vi "Quaternion_ToRotationVector.vi"(11 "Quaternion":T1={"R"=1.0, "V"=[0.0, 0.0, 0.0]}) -> (3 "RotationVector":dbl[](array[numeric]))   [LabVIEW 2019, in "Trajectory_Library.lvlib"]
doc: "Returns the rotation vector representation of this quaternion.\n\nThis is also the log operator of SO(3).\n\nParameters:\n - Quaternion -- The quaternion data cluster.\n\nReturns:\n - Rotation Vector - The rotation vector representation of this quaternion."
uses:
  Trajectory_Library.lvlib
  TypeDef/QUATERNION.ctl
  <vilib>/Analysis/_algsub.llb/Matrix Norm.vi
  <vilib>/Analysis/_algsub.llb/Real Matrix Norm.vi
  <vilib>/Analysis/Matrix/Numeric/Conversions/Array To Matrix - RA.vi
  <vilib>/Analysis/Matrix/NI_Matrix.lvlib
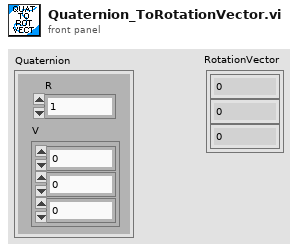
[diagram p1: front panel]
types:
  T1 = typedef "Trajectory_Library.lvlib/QUATERNION.ctl" = cluster{"R":dbl, "V":dbl[]}
  T2 = typedef "NI_Matrix.lvlib/RealMatrix.ctl" = dbl[][]
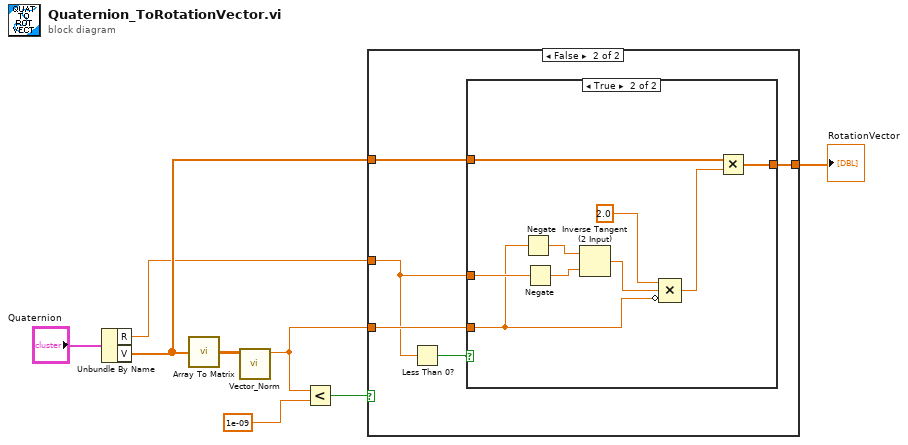
[diagram p0: block diagram]
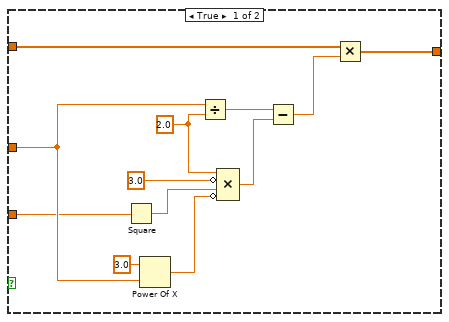
[diagram p2: hidden frame]
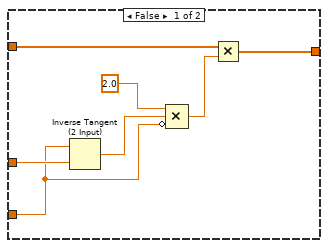
[diagram p3: hidden frame]
diagram:
  n1 = Unbundle By Name("Quaternion") -> ("R"=w3:dbl, "V"=w5:dbl[])
  n2 = call-poly <vilib>:"Array To Matrix.vi"("Real 1D Array"=w5) -> ("Real Matrix (Column Vector)"=w2:T2)
  n3 = call "Vector_Norm.vi"("Input Vector"=w2) -> ("norm"=w1:dbl)  [unwired: 10 in]
  n4 = Less?(x=w1, y=1e-09) -> (x < y?=w6:bool)
  n5 = case shown="False" w6 {
    tunnel: w5 -> [w20 w24]
    tunnel: [w19 w23] -> w4
    tunnel: w3 -> [w17 w21]
    tunnel: w1 -> [w16 w22]
    frame True {
      w15 = 2.0 ("y")
      n6 = Square(x=w16) -> (x^2=w13:dbl)
      n7 = Power Of X(1:w17, 2:3.0 ("y")) -> (0:w12:dbl)
      n8 = Divide(x=w17, y=w15) -> (x/y=w11:dbl)
      n9 = Compound Arithmetic op=MULTIPLY(w15, invert 3.0 ("y"), w13, invert w12) -> (w10:dbl)
      n10 = Subtract(x=w11, y=w10) -> (x-y=w9:dbl)
      n11 = Multiply(x=w20, y=w9) -> (x*y=w19:dbl[])
    }
    frame False {
      n12 = Less Than 0?(x=w21) -> (x < 0?=w25:bool)
      n13 = case shown="True" w25 {
        tunnel: w24 -> [w29 w40]
        tunnel: [w30 w39] -> w23
        tunnel: w22 -> [w26 w33]
        tunnel: w21 -> [w27 w36]
        frame False {
          n14 = Inverse Tangent (2 Input)(1:w27, 2:w26) -> (0:w31:dbl)
          n15 = Compound Arithmetic op=MULTIPLY(2.0 ("y"), w31, invert w26) -> (w28:dbl)
          n16 = Multiply(x=w29, y=w28) -> (x*y=w30:dbl[])
        }
        frame True {
          n17 = Negate(x=w33) -> (-x=w37:dbl)
          n18 = Negate(x=w36) -> (-x=w35:dbl)
          n19 = Inverse Tangent (2 Input)(1:w35, 2:w37) -> (0:w34:dbl)
          n20 = Compound Arithmetic op=MULTIPLY(2.0 ("y"), w34, invert w33) -> (w38:dbl)
          n21 = Multiply(x=w40, y=w38) -> (x*y=w39:dbl[])
        }
      }
    }
  }
  "RotationVector" <- w4
